vi "PD Detection Display 3.vi"() -> ()   [LabVIEW 2013]
uses:
  <vilib>/Instr/_visa.llb/VISA Open Access Mode.ctl
  <vilib>/Instr/_visa.llb/VISA Flush IO Buffer Mask.ctl
  <vilib>/Instr/_visa.llb/VISA Configure Serial Port (Instr).vi
  <vilib>/Utility/file.llb/Write To Spreadsheet File (DBL).vi
panel:
  in  "VISA resource name":refnum<visa-resource-name>="COM4"
  in  "Notes":string="data"
  in  "Save Histogram?":bool=TRUE
  in  "Num Samples":u64=10000
  in  "Samples":bool
  out "PD/s (now)":dbl
  out "Bytes at Port":u32
  out "PD/s (total)":dbl
  out "raw data":string
  out "Waveform Chart":dbl[](graph)
  out "array":dbl[](array[numeric])
  out "Packets at Port":u32
  in  "stop":bool
  # "Infinite"
  # "This Many ->"
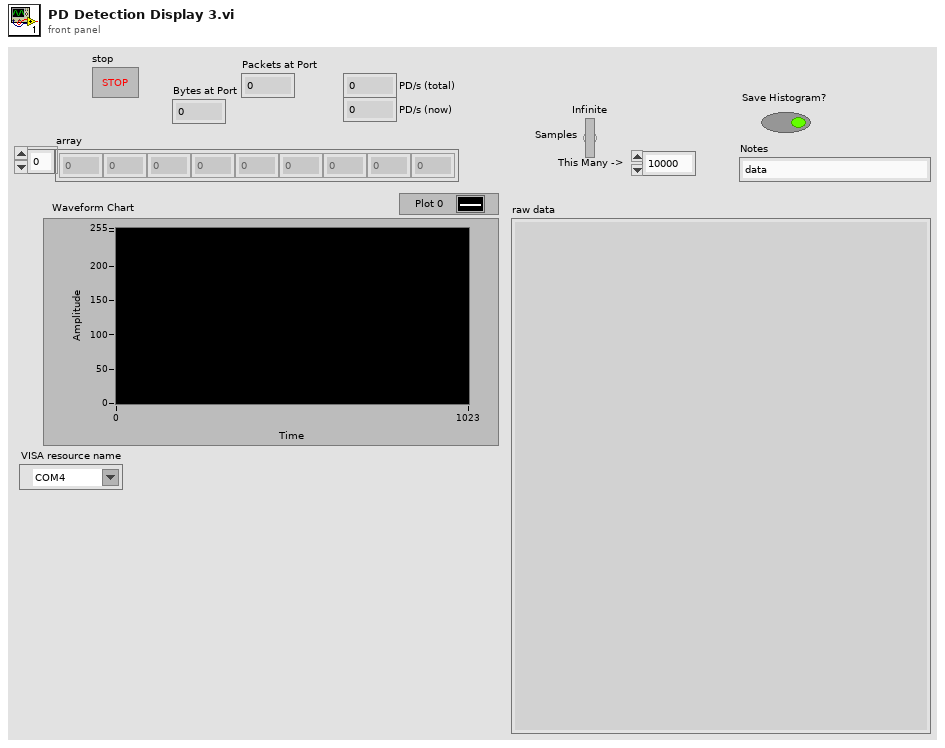
[diagram p1: front panel]
types:
  T1 = typedef "VISA Flush IO Buffer Mask.ctl" = u16
  T2 = typedef "VISA Open Access Mode.ctl" = u32
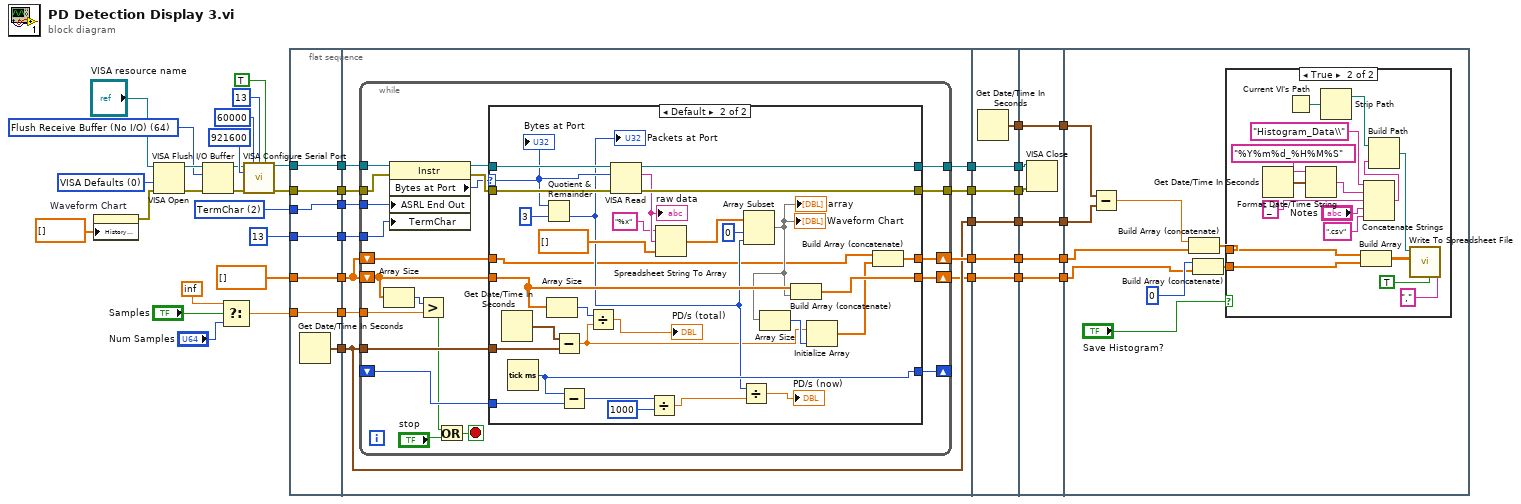
[diagram p0: block diagram]
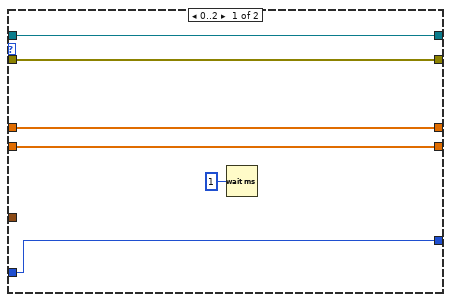
[diagram p2: hidden frame]
diagram:
  w12 = u16 2 items=["None", "Last Bit", "TermChar", "Break"] ("Serial Settings:End Mode for Writes")
  w34 = T1 64 items=["Flush Receive Buffer"=16, "Write Transmit Buffer to Device"=32, "Flush Receive Buffer (No I/O)"=64, "Flush Transmit Buffer"=128] ("Mask")
  w41 = T2 0 items=["VISA Defaults"=0, "Exclusive Lock"=1, "Load Configured Settings"=4] ("Access Mode")
  n1 = property on="Waveform Chart" class="WFChart (strict)"("History Data"=dbl[] []) -> (error out=w33:errorcluster)  [unwired: 2 in, 1 out]
  n2 = VISA Open(access mode=w41, error in (no error)=w33, VISA resource name="VISA resource name") -> (VISA resource name=w37:refnum<visa-resource-name>, error out=w38:errorcluster)  [unwired: 2 in]
  n3 = VISA Flush I/O Buffer(VISA resource name=w37, mask (16)=w34, error in (no error)=w38) -> (VISA resource name out=w35:refnum<visa-resource-name>, error out=w36:errorcluster)
  n4 = Select(t=inf, s="Samples", f="Num Samples") -> (s? t:f=w5:dbl)
  n5 = call-poly "VISA Configure Serial Port"("VISA resource name"=w35, "timeout (10sec)"=u32 60000, "termination char\n(0xA = '\\n' = LF)"=u8 13 ("termination char\n(0xA = '\\n' = LF)"), "Enable Termination\nChar (T)"=TRUE ("Enable Termination\nChar (T)"), "baud rate (9600)"=u32 921600, "error in (no error)"=w36) -> ("VISA resource name out"=w15:refnum<visa-resource-name>, "error out"=w14:errorcluster)  [unwired: 8 in]
  n6 = flat-sequence {
    tunnel: [w51] -> w17
    tunnel: [w50] -> w16
    tunnel: w15 -> [w50]
    tunnel: w14 -> [w49]
    tunnel: [w49] -> w13
    tunnel: w12 -> [w48]
    tunnel: [w48] -> w11
    tunnel: u8 13 ("termination char\n(0xA = '\\n' = LF)") -> [w47]
    tunnel: [w47] -> w9
    tunnel: dbl[] [] -> [w46]
    tunnel: [w46] -> w7
    tunnel: [w45] -> w6
    tunnel: w5 -> [w45]
    tunnel: [w60] -> w20
    tunnel: [w62] -> w19
    tunnel: [w61] -> w18
    tunnel: w17 -> [w54]
    tunnel: w16 -> [w59]
    tunnel: w13 -> [w58]
    tunnel: w11 -> [w57]
    tunnel: w9 -> [w56]
    tunnel: w7 -> [w53]
    tunnel: w6 -> [w55]
    tunnel: [w54] -> w4
    tunnel: [w52] -> w1
    tunnel: [w125] -> w26
    tunnel: [w124] -> w25
    tunnel: [w123] -> w23
    tunnel: [w122] -> w22
    tunnel: [w121] -> w21
    tunnel: w20 -> [w125]
    tunnel: w19 -> [w122]
    tunnel: w18 -> [w121]
    tunnel: w4 -> [w124]
    tunnel: [w120] -> w2
    tunnel: w1 -> [w120]
    tunnel: [w131] -> w28
    tunnel: [w130] -> w27
    tunnel: w26 -> [w131]
    tunnel: w25 -> [w130]
    tunnel: [w129] -> w24
    tunnel: w23 -> [w129]
    tunnel: w22 -> [w128]
    tunnel: w21 -> [w127]
    tunnel: [w126] -> w3
    tunnel: w2 -> [w126]
    tunnel: w28 -> [w132]
    tunnel: w27 -> [w139]
    tunnel: w24 -> [w134]
    tunnel: w3 -> [w133]
    frame #0 {
      n7 = Get Date/Time In Seconds() -> (seconds since 1Jan1904=w51:timestamp)
    }
    frame #1 {
      n8 = while {
        tunnel: [w83] -> w61
        tunnel: [w82] -> w62
        tunnel: w59 -> [w78]
        tunnel: w58 -> [w79]
        shift-right: [w81] -> w52
        shift-left: w53 -> [w70]
        tunnel: w54 -> [w80]
        tunnel: w57 -> [w74]
        tunnel: w56 -> [w73]
        shift-right: [w72] -> _
        shift-left: _ -> [w71]
        tunnel: w55 -> [w69]
        shift-right: [w64] -> w60
        shift-left: w53 -> [w63]
        stop <- w67 stop-if-true
        n9 = Array Size(array=w70) -> (size(s)=w68:i32)
        n10 = property class="Instr"(reference=w78, error in=w79, "ASRL End Out"=w74, "TermChar"=w73) -> (reference out=w77:refnum<visa-resource-name>, error out=w76:errorcluster, "Bytes at Port"=w75:u32)
        n11 = Greater?(x=w68, y=w69) -> (0:w66:bool)
        n12 = Or(x=w66, y="stop") -> (x .or. y?=w67:bool)
        n13 = case shown="Default" w75 {
          selector: w75 -> [_ w100]
          tunnel: [w88 w118] -> w83
          tunnel: [w89 w117] -> w82
          tunnel: w76 -> [w88 w119]
          tunnel: w77 -> [w89 w116]
          tunnel: [w87 w112] -> w81
          tunnel: w70 -> [w87 w111]
          tunnel: w80 -> [_ w109]
          tunnel: [w85 w104] -> w72
          tunnel: w71 -> [w85 w106]
          tunnel: [w84 w90] -> w64
          tunnel: w63 -> [w84 w91]
          frame 0..2 {
            n14 = Wait (ms)(milliseconds to wait=u32 1) -> ()  [unwired: 1 out]
          }
          frame Default {
            n15 = Get Date/Time In Seconds() -> (seconds since 1Jan1904=w107:timestamp)
            n16 = Tick Count (ms)() -> (millisecond timer value=w104:u32)
            n17 = Quotient & Remainder(x=w100, y=u32 3) -> (floor(x/y)=w97:u32)  [unwired: 1 out]
            "Packets at Port" <- w97
            n18 = Array Size(array=w111) -> (size(s)=w110:i32)
            n19 = Subtract(x=w107, y=w109) -> (x-y=w93:dbl)
            n20 = Subtract(x=w104, y=w106) -> (x-y=w103:u32)
            n21 = Divide(x=w110, y=w93) -> (x/y=→"PD/s (total)":dbl)
            n22 = VISA Read(VISA resource name=w116, byte count=w100, error in (no error)=w119) -> (VISA resource name out=w117:refnum<visa-resource-name>, read buffer=w114:string, error out=w118:errorcluster)  [unwired: 1 out]
            "raw data" <- w114
            n23 = Divide(x=w103, y=u32 1000) -> (x/y=w102:dbl)
            n24 = Spreadsheet String To Array(format string="%x", spreadsheet string=w114, array type (2D Dbl)=dbl[] []) -> (array=w98:dbl[])  [unwired: 1 in]
            n25 = Divide(x=w97, y=w102) -> (x/y=→"PD/s (now)":dbl)
            n26 = Array Subset(array=w98, index=0, length=w97) -> (w95:dbl[])
            "array" <- w95
            "Waveform Chart" <- w95
            n27 = Array Size(array=w95) -> (size(s)=w94:i32)
            n28 = Build Array (concatenate)(w111, w95) -> (w112:dbl[])
            n29 = Initialize Array(w93, w94) -> (w92:dbl[])
            n30 = Build Array (concatenate)(w91, w92) -> (w90:dbl[])
            "Bytes at Port" <- w100
          }
        }
      }
    }
    frame #2 {
      n31 = Get Date/Time In Seconds() -> (seconds since 1Jan1904=w123:timestamp)
    }
    frame #3 {
      n32 = VISA Close(VISA resource name=w128, error in (no error)=w127) -> ()  [unwired: 1 out]
    }
    frame #4 {
      n33 = Subtract(x=w134, y=w139) -> (x-y=w137:dbl)
      n34 = Build Array (concatenate)(w137, w132) -> (w136:dbl[])
      n35 = Build Array (concatenate)(0, w133) -> (w138:dbl[])
      n36 = case shown="True" "Save Histogram?" {
        tunnel: w136 -> [_ w142]
        tunnel: w138 -> [_ w141]
        frame False {
        }
        frame True {
          n37 = Get Date/Time In Seconds() -> (seconds since 1Jan1904=w155:timestamp)
          n38 = Current VI's Path() -> (path=w151:path)
          n39 = Format Date/Time String(time format string (%c)="%Y%m%d_%H%M%S", seconds (now)=w155) -> (date/time string=w152:string)  [unwired: 1 in]
          n40 = Strip Path(path=w151) -> (stripped path=w150:path)  [unwired: 1 out]
          n41 = Build Array(w142, w141) -> (w156:dbl[][])
          n42 = Concatenate Strings("Histogram_Data\\", w152, "_", "Notes", ".csv") -> (w149:string)
          n43 = Build Path(base path=w150, name or relative path=w149) -> (appended path=w148:path)
          n44 = call-poly <vilib>:"Write To Spreadsheet File.vi"("delimiter (\\t)"="," ("delimiter (\\t)"), "transpose? (no:F)"=TRUE, "2D data"=w156, "file path (dialog if empty)"=w148) -> ()  [unwired: 4 in, 1 out]
        }
      }
    }
  }
